vi "NKT_Config.vi"(8 "entrée d'erreur (pas d'erreur)":errorcluster) -> (0 "sortie d'erreur":errorcluster)   [LabVIEW 2026]
doc: "+--------------------------------------------------------------+\n¦ ÉTAT CONFIG ¦\n¦ ¦\n¦ 1. RegisterWriteU8 — Emission ¦\n¦ PortName : portName (shift register) ¦\n¦ DeviceID : 15 | RegID : 48 | Index : -1 ¦\n¦ Value U8 : cluster ON/OFF ? 3 si TRUE, 0 si FALSE ¦\n¦ ¦\n¦ 2. RegisterWriteU16 — Puissance ¦\n¦ PortName : portName (shift register) ¦\n¦ DeviceID : 15 | RegID : 55 | Index : -1 ¦\n¦ Value U16 : cluster Power × 10 ¦\n¦ ¦\n¦ 3. RegisterWriteU16 — LWP ¦\n¦ PortName : portName (shift register) ¦\n¦ DeviceID : 16 | RegID : 52 | Index : -1 ¦\n¦ Value U16 : Floor(Lambda - Bandwidth/2) × 10 ¦\n¦ ¦\n¦ 4. RegisterWriteU16 — SWP ¦\n¦ PortName : portName (shift register) ¦\n¦ DeviceID : 16 | RegID : 51 | Index : -1 ¦\n¦ Value U16 : Floor(Lambda + Bandwidth/2) × 10 ¦\n¦ ¦\n¦ 5. RegisterWriteU16 — ND ¦\n¦ PortName : portName (shift register) ¦\n¦ DeviceID : 16 | RegID : 32 | Index : -1 ¦\n¦ Value U16 : cluster ND × 10 ¦\n+---------------------------------------------------------------+"
uses:
  Controls/TypeDef_FGV.ctl
  <instrlib>/NKTP_API/NKTP_API.lvlib
panel:
  out "floor(x) : plus grand entier <= x":dbl
  out "portname out":string
  out "ID":i32 caption="Numérique"
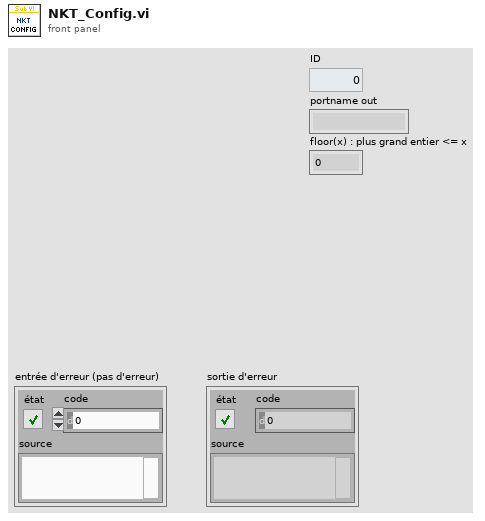
[diagram p1: front panel]
types:
  T1 = typedef "TypeDef_FGV.ctl" = enum16{"Initialize", "Write", "Read"}
  T2 = typedef "Laser.ctl" = cluster{"Emission (ON/OFF)":bool, "Wavelength (nm)":dbl, "Bandwidth (nm)":dbl, "Power (%)":dbl, "ND (%)":dbl}
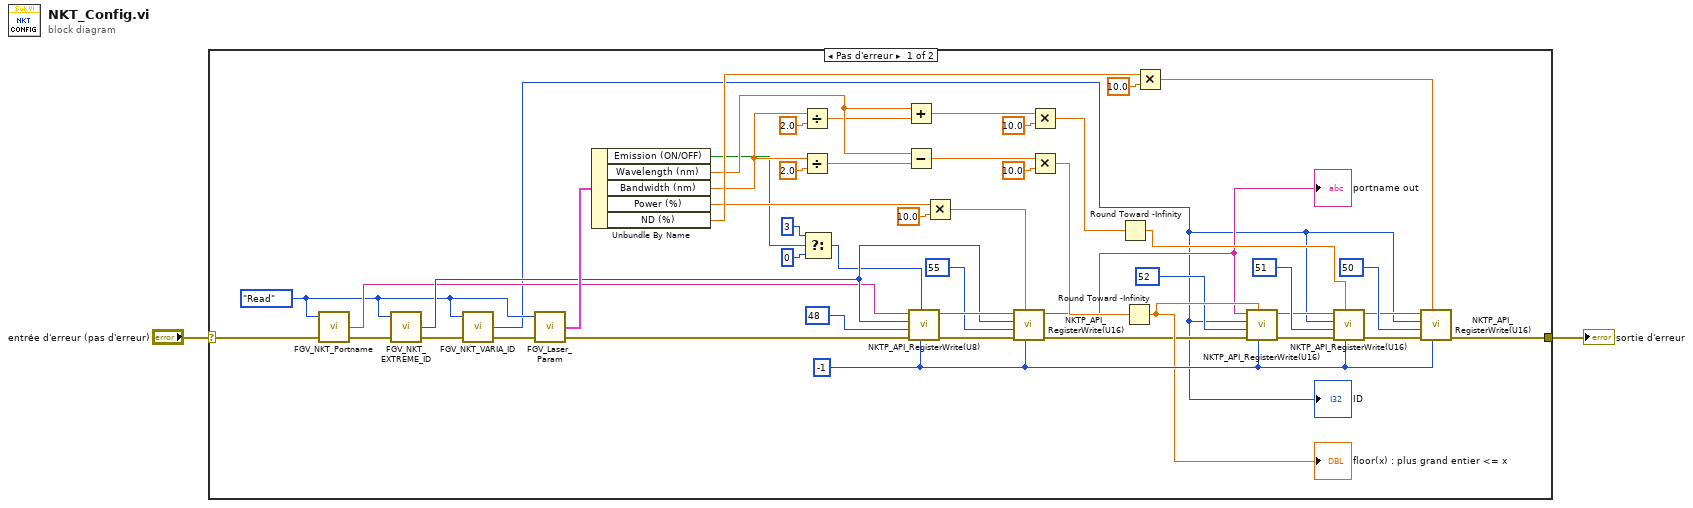
[diagram p0: block diagram]
diagram:
  n1 = case shown="Pas d'erreur" "entrée d'erreur (pas d'erreur)" {
    selector: "entrée d'erreur (pas d'erreur)" -> [w13 w52]
    tunnel: [w49 w52] -> w2
    frame No Error {
      w50 = i16 -1 ("index")
      w10 = TypeDef_FGV."Read" ("Action")
      n2 = call "FGV_NKT_Portname.vi"("error in"=w13, "Action"=w10) -> ("error out"=w12:errorcluster, "Portname"=w11:string)  [unwired: 2 in]
      n3 = call "FGV_NKT_EXTREME_ID.vi"("error in"=w12, "Action"=w10) -> ("error out"=w15:errorcluster, "ID"=w14:i32)  [unwired: 2 in]
      n4 = call "FGV_NKT_VARIA_ID.vi"("error in"=w15, "Action"=w10) -> ("error out"=w16:errorcluster, "ID"=w3:i32)  [unwired: 2 in]
      "ID" <- w3
      n5 = call "FGV_Laser_Param.vi"("error in"=w16, "Action"=w10) -> ("error out"=w18:errorcluster, "Laser params"=w17:T2)  [unwired: 2 in]
      n6 = Unbundle By Name(w17) -> ("Emission (ON/OFF)"=w8:bool, "Wavelength (nm)"=w40:dbl, "Bandwidth (nm)"=w41:dbl, "Power (%)"=w9:dbl, "ND (%)"=w46:dbl)
      n7 = Divide(x=w41, y=2.0) -> (x/y=w39:dbl)
      n8 = Divide(x=w41, y=2.0) -> (x/y=w27:dbl)
      n9 = Select(t=u8 3 ("cas vrai"), s=w8, f=u8 0 ("cas faux")) -> (s? t:f=w7:u8)
      n10 = Add(x=w40, y=w39) -> (x+y=w37:dbl)
      n11 = Subtract(x=w40, y=w27) -> (x-y=w29:dbl)
      n12 = call <instrlib>:"NKTP_API_RegisterWrite(U8).vi"("index"=w50, "value"=w7, "error in"=w18, "regId"=u8 48, "devId"=w14, "portname"=w11) -> ("error out"=w21:errorcluster, "portname out"=w20:string)  [unwired: 4 in]
      n13 = Multiply(x=w9, y=10.0) -> (x*y=w22:dbl)
      n14 = call <instrlib>:"NKTP_API_RegisterWrite(U16).vi"("index"=w50, "value"=w22, "error in"=w21, "regId"=u8 55, "devId"=w14, "portname"=w20) -> ("error out"=w25:errorcluster, "portname out"=w24:string)  [unwired: 4 in]
      "portname out" <- w24
      n15 = Multiply(x=w37, y=10.0) -> (x*y=w35:dbl)
      n16 = Multiply(x=w29, y=10.0) -> (x*y=w31:dbl)
      n17 = Round Toward -Infinity(1:w35) -> (0:w42:dbl)
      n18 = Round Toward -Infinity(1:w31) -> (0:w32:dbl)
      "floor(x) : plus grand entier <= x" <- w32
      n19 = Multiply(x=w46, y=10.0) -> (x*y=w47:dbl)
      n20 = call <instrlib>:"NKTP_API_RegisterWrite(U16).vi"("index"=w50, "value"=w32, "error in"=w25, "regId"=u8 52, "devId"=w3, "portname"=w24) -> ("error out"=w34:errorcluster, "portname out"=w33:string)  [unwired: 4 in]
      n21 = call <instrlib>:"NKTP_API_RegisterWrite(U16).vi"("index"=w50, "value"=w42, "error in"=w34, "regId"=u8 51, "devId"=w3, "portname"=w33) -> ("error out"=w45:errorcluster, "portname out"=w44:string)  [unwired: 4 in]
      n22 = call <instrlib>:"NKTP_API_RegisterWrite(U16).vi"("index"=w50, "value"=w47, "error in"=w45, "regId"=u8 50, "devId"=w3, "portname"=w44) -> ("error out"=w49:errorcluster)  [unwired: 4 in, 1 out]
    }
    frame Error {
    }
  }
  "sortie d'erreur" <- w2
